vi "MetaClientSendOk.vi"(8 "error in (no error)":errorcluster) -> (3 "Boolean":bool)   [LabVIEW 2017]
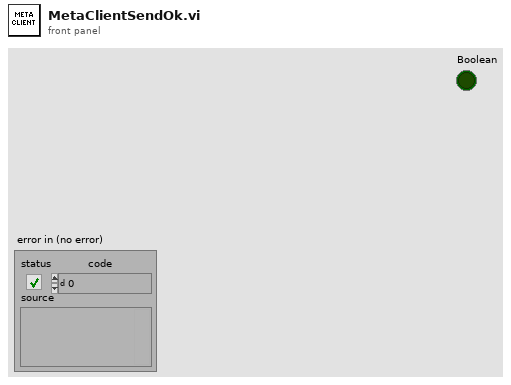
[diagram p1: front panel]
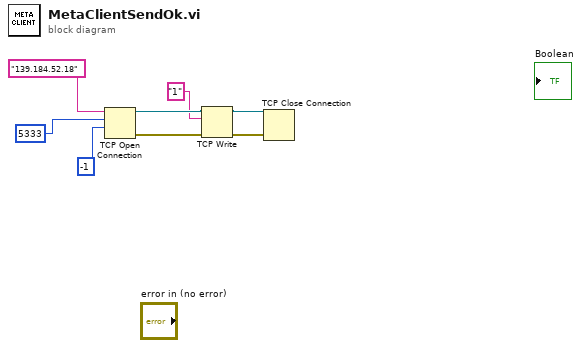
[diagram p0: block diagram]
diagram:
  n1 = TCP Open Connection(address="139.184.52.18", remote port or service name=u16 5333, timeout ms (60000)=-1) -> (connection ID=w3:refnum<k5>, error out=w2:errorcluster)  [unwired: 2 in]
  n2 = TCP Write(connection ID=w3, data in="1", error in (no error)=w2) -> (connection ID out=w5:refnum<k5>, error out=w4:errorcluster)  [unwired: 1 in, 1 out]
  n3 = TCP Close Connection(connection ID=w5, error in (no error)=w4) -> ()  [unwired: 1 in, 2 out]
